vi "gade-delay.vi"(9 "reset value":bool, 10 "delay":i16, 11 "total count":i16) -> (3 "x > y?":bool)   [LabVIEW 2018]
uses:
  <vilib>/rvi/Emulation/niFpgaGetClockAttributes.vi
  <vilib>/rvi/Emulation/niFpgaSctlEmulationGetInTimedLoop.vi
  <vilib>/rvi/Emulation/niFpgaEmulationReportErrorSimple.vi
  <vilib>/rvi/Emulation/niFpgaCriticalErrorInLSC.vi
  <vilib>/Platform/TimedLoop/XDataNode/timing_clust.ctl
  <vilib>/Platform/TimedLoop/XDataNode/wakeup.ctl
  <vilib>/Platform/TimedLoop/XDataNode/nitl_modes.ctl
  <vilib>/eio/EIONode/EIONode.xnode
  <vilib>/rvi/eio/common/nirviEmuTemplateMethod_errors.vi
  <vilib>/Platform/TimedLoop/XDataNode/XDataNode.xnode
  <vilib>/Platform/TimedLoop/XDataNode/XDNodeRunTimeDep.lvlib
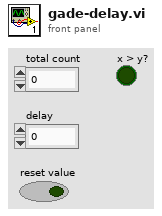
[diagram p1: front panel]
types:
  T1 = typedef "XDNodeRunTimeDep.lvlib/timing_clust.ctl" = cluster{"Expected End [f-1]":u64, "Actual End [f-1]":u64, "Finished Late? [f-1]":bool, "Expected End [i-1]":u64, "Actual End [i-1]":u64, "Finished Late? [i-1]":bool, "Expected Start [i]":u64, "Actual Start [i]":u64, "Expected Start [f]":u64, "Actual Start [f]":u64, "Source Name":string, "Structure Name":string, "Period":i64, "Deadline":i64, "Offset":i64, "Start":i64, "Priority":i32, "Timeout":i32, "Mode":T2, "Wakeup Reason":T3, "Error":errorcluster, "Source Type":string, "Secondary Source Type":string, "Global End Time":u64, "Global Start Time":u64, "Frame Duration":u64, "Iteration Duration":u64, "Assigned CPU":i32, "I/O Scan Engine Mode":u32}
  T2 = typedef "XDNodeRunTimeDep.lvlib/nitl_modes.ctl" = enum32{"No Change", "Process missed periods, maintain original phase", "Discard missed periods, maintain original phase", "Process missed periods, ignore original phase", "Discard missed periods, ignore original phase"}
  T3 = typedef "XDNodeRunTimeDep.lvlib/wakeup.ctl" = enum32{"Normal", "Aborted", "Asynchronous wakeup", "Timing source error", "Timed loop error", "Timeout"}
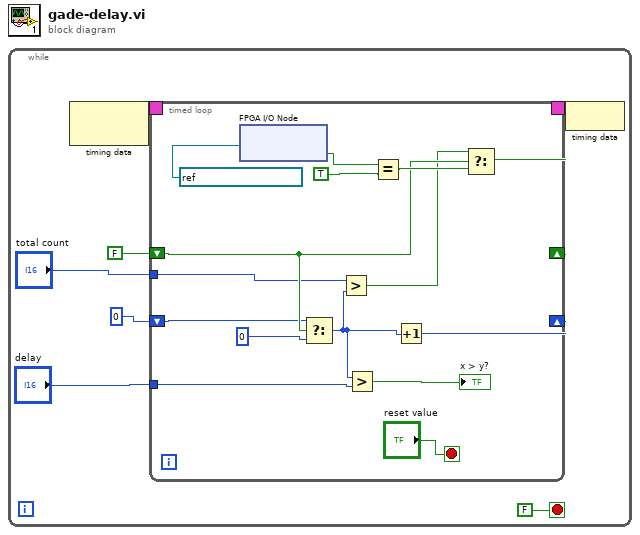
[diagram p0: block diagram]
diagram:
  n1 = while {
    stop <- FALSE stop-if-true
    n2 = node-c288() -> (w7:T1)  [unwired: 1 in]
    n3 = timed-loop {
      timing: w7 -> [_]
      timing-out: [_] -> w6
      shift-right: [w22] -> _
      shift-left: FALSE -> [w17]
      shift-right: [w19] -> _
      shift-left: i16 0 -> [w16]
      tunnel: "total count" -> [w15]
      tunnel: "delay" -> [w13]
      stop <- "reset value" stop-if-true
      n4 = xnode "FPGA I/O Node"("FPGA I/O In"=refnum<k21> "ConnectorA/DIO0") -> ("I/O Item"=w9:bool)  [unwired: 1 out]
      n5 = Select(t=w16, s=w17, f=i16 0) -> (s? t:f=w12:i16)
      n6 = Greater?(x=w15, y=w12) -> (0:w14:bool)
      n7 = Greater?(x=w12, y=w13) -> (0:→"x > y?":bool)
      n8 = Equal?(x=w9, y=TRUE) -> (x = y?=w20:bool)
      n9 = Increment(x=w12) -> (x+1=w19:i16)
      n10 = Select(t=w14, s=w17, f=w20) -> (s? t:f=w22:bool)
    }
    n11 = node-c288(w6) -> ()
  }
